vi "HDI Pat Match Full with Move TL.vi"(5 "controller in":refnum<k24>, 11 "error in":errorcluster) -> (4 "In Range?":bool, 8 "x rel move":dbl, 10 "y rel move":dbl, 14 "Vertical vector":dbl[](array[numeric]), 15 "error out":errorcluster)   [LabVIEW 2011]
uses:
  C:/Users/Admin/Desktop/Gantry Code Transfer/source/Code Transfer/Aerotech.A3200.dll
  Aerotech.A3200.dll
  <vilib>/vision/driver/NI_Vision_Acquisition_Software.lvlib
panel:
  out "error out 3":errorcluster
  out "error out 2":errorcluster
  out "Angle Between Lines":dbl
  out "Diagnostic Log":string
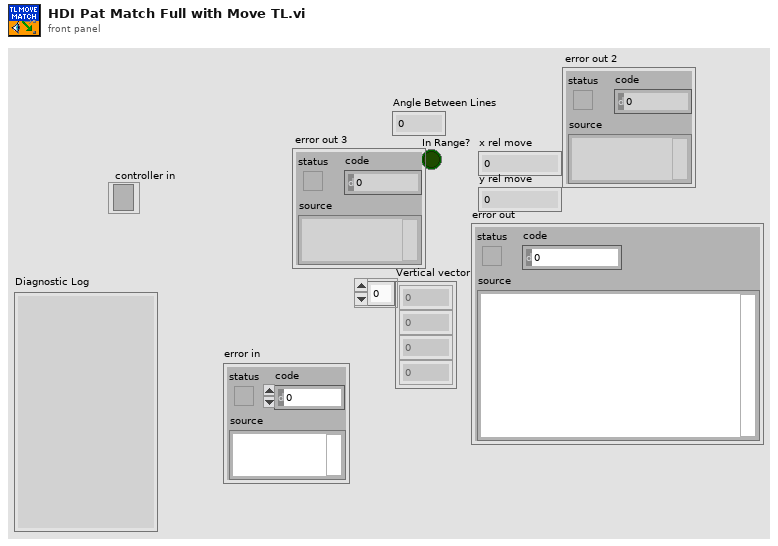
[diagram p1: front panel]
types:
  T1 = typedef "IMAQdx.ctl" = refnum<k21>
  T2 = typedef "IMAQ Image.ctl" = refnum<image>
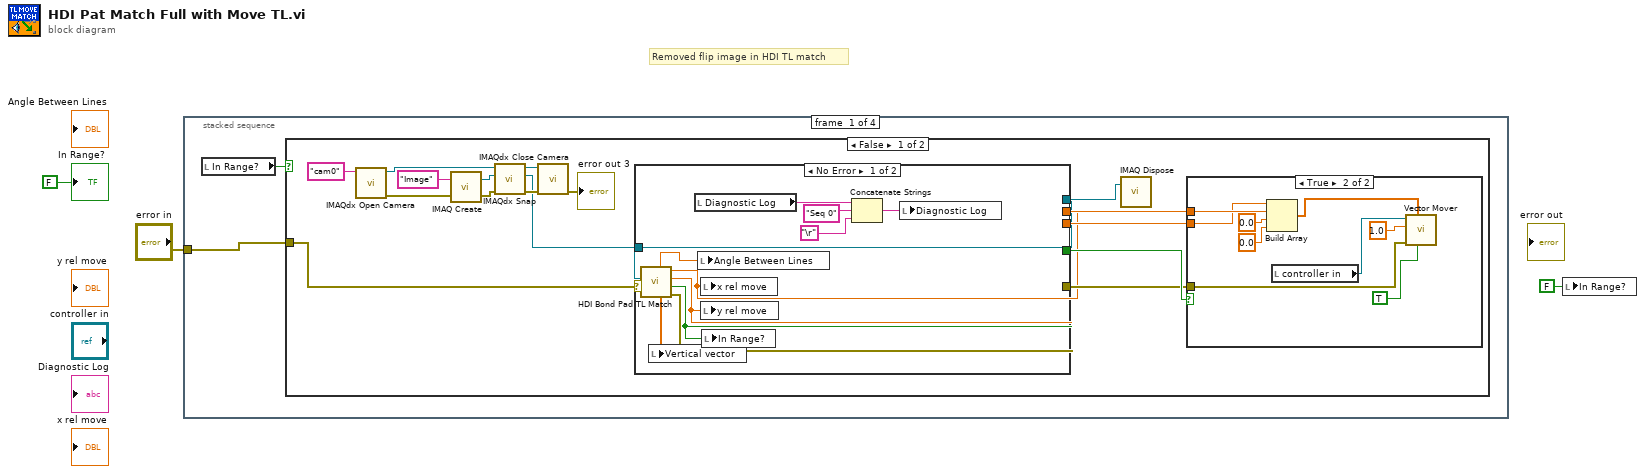
[diagram p0: block diagram]
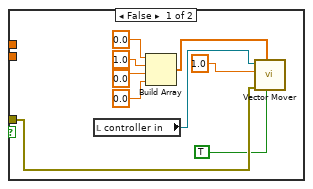
[diagram p2: hidden frame]
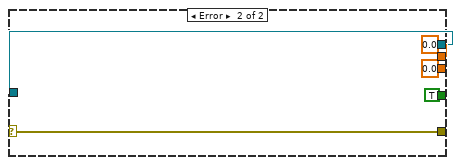
[diagram p3: hidden frame]
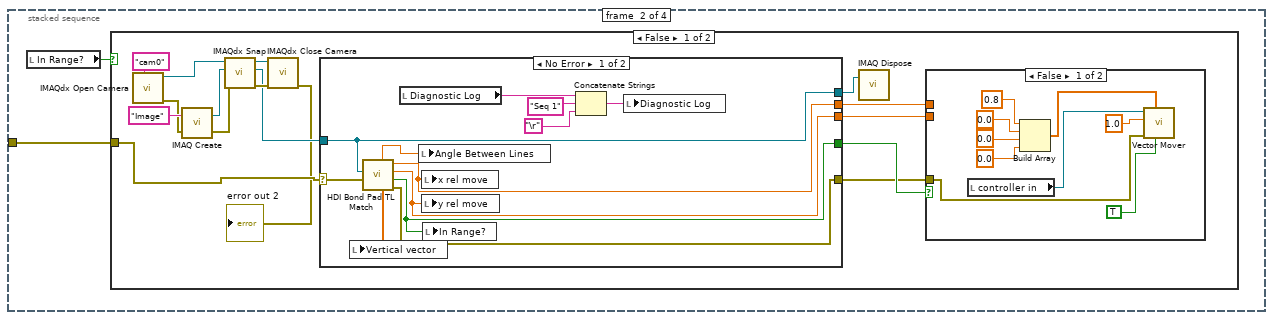
[diagram p5: hidden frame]
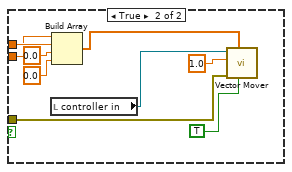
[diagram p6: hidden frame]
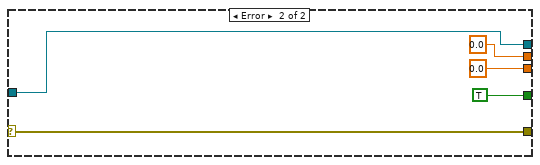
[diagram p7: hidden frame]
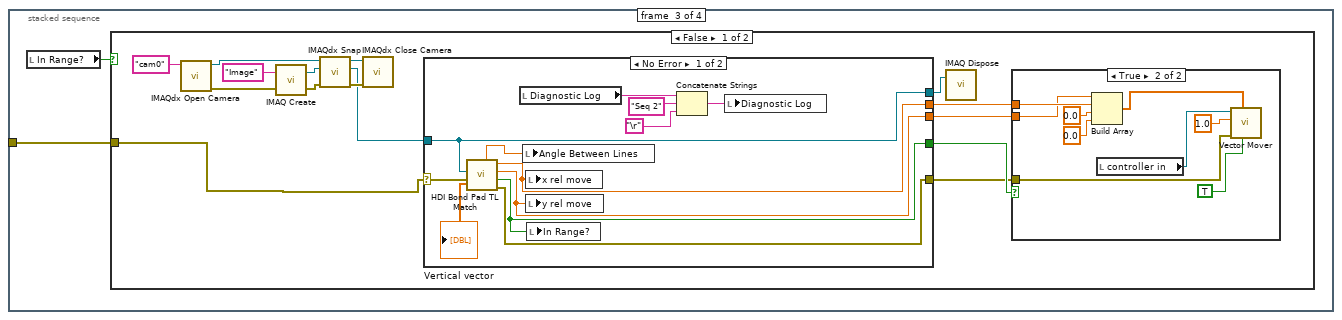
[diagram p9: hidden frame]
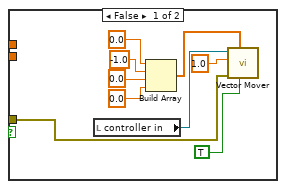
[diagram p10: hidden frame]
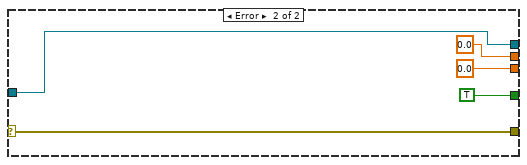
[diagram p11: hidden frame]
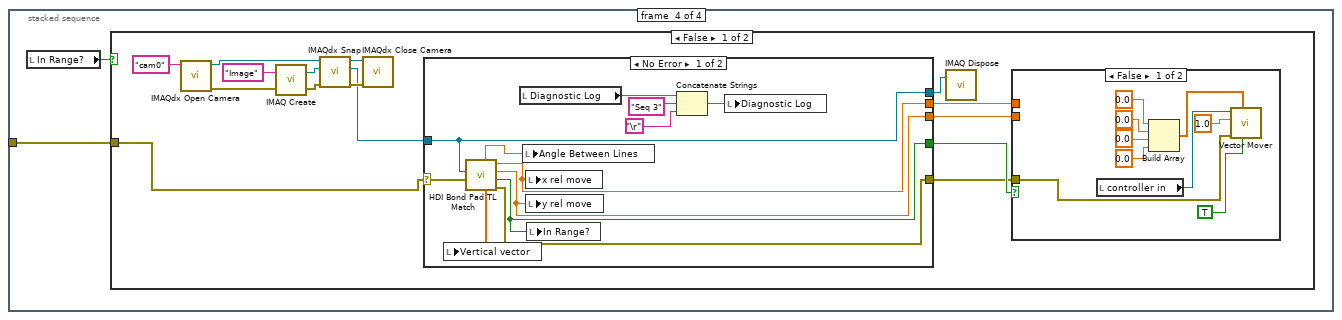
[diagram p13: hidden frame]
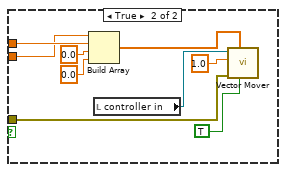
[diagram p14: hidden frame]
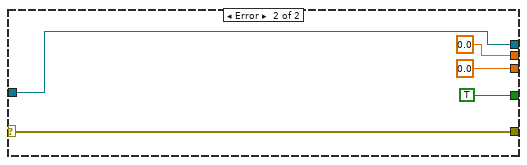
[diagram p15: hidden frame]
diagram:
  # "Removed flip image in HDI TL match"
  n1 = stacked-sequence {
    tunnel: "error in" -> [w4 w57 w110 w162]
    frame #0 {
      n2 = local read "In Range?"() -> (w5:bool)
      n3 = case shown="False" w5 {
        tunnel: w4 -> [w7 _]
        frame False {
          n4 = call <vilib>:"IMAQdx Open Camera.vi"("Session In"="cam0" ("Interface Name")) -> ("error out"=w14:errorcluster, "Session Out"=w9:T1)  [unwired: 9 in]
          n5 = call "IMAQ Create"("Image Name"="Image", "error in (no error)"=w14) -> ("New Image"=w11:T2, "error out"=w10:errorcluster)  [unwired: 3 in]
          n6 = call <vilib>:"IMAQdx Snap.vi"("error in"=w10, "Image In"=w11, "Session In"=w9) -> ("error out"=w12:errorcluster, "Image Out"=w8:T2, "Session Out"=w13:T1)  [unwired: 6 in]
          n7 = call <vilib>:"IMAQdx Close Camera.vi"("error in"=w12, "Session In"=w13) -> ("error out"=→"error out 3":errorcluster)  [unwired: 9 in]
          n8 = case shown="No Error" w7 {
            selector: w7 -> [w50 w56]
            tunnel: [w51 w56] -> w20
            tunnel: [w47 TRUE ("Matched?")] -> w21
            tunnel: [w49 0.0 ("x rel move")] -> w19
            tunnel: [w48 0.0 ("y rel move")] -> w18
            tunnel: w8 -> [w42 w52]
            tunnel: [w42 w52] -> w17
            frame No Error {
              n9 = call "HDI Bond Pad TL Match.vi"("error in (no error)"=w50, "Image Src"=w42) -> ("error out"=w51:errorcluster, "In Range?"=w47:bool, "y rel move"=w48:dbl, "x rel move"=w49:dbl, "Vertical vector"=w40:dbl[], "Angle Between Lines"=w41:dbl)  [unwired: 4 in]
              n10 = local write "Vertical vector"(w40) -> ()
              n11 = local read "Diagnostic Log"() -> (w43:string)
              n12 = local write "Angle Between Lines"(w41) -> ()
              n13 = local write "x rel move"(w49) -> ()
              n14 = local write "y rel move"(w48) -> ()
              n15 = local write "In Range?"(w47) -> ()
              n16 = Concatenate Strings(w43, "Seq 0", "\r") -> (w46:string)
              n17 = local write "Diagnostic Log"(w46) -> ()
            }
            frame Error {
            }
          }
          n18 = call "IMAQ Dispose"("Image"=w17) -> ()  [unwired: 5 in, 1 out]
          n19 = case shown="True" w21 {
            tunnel: w20 -> [w25 w39]
            tunnel: w19 -> [_ w32]
            tunnel: w18 -> [_ w31]
            frame False {
              n20 = local read "controller in"() -> (w24:refnum<k24>)
              n21 = Build Array(0.0 ("element"), 1.0 ("element"), 0.0 ("element"), 0.0 ("element")) -> (w23:dbl[])
              n22 = call "Vector Mover.vi"("Absolute/Relative (F/T)"=TRUE, "Movement Vector"=w23, "error in (no error)"=w25, "Vector Speed"=1.0, "controller in"=w24) -> ()  [unwired: 1 in, 4 out]
            }
            frame True {
              n23 = Build Array(w31, w32, 0.0 ("element"), 0.0 ("element")) -> (w34:dbl[])
              n24 = local read "controller in"() -> (w33:refnum<k24>)
              n25 = call "Vector Mover.vi"("Absolute/Relative (F/T)"=TRUE, "Movement Vector"=w34, "error in (no error)"=w39, "Vector Speed"=1.0, "controller in"=w33) -> ()  [unwired: 1 in, 4 out]
            }
          }
        }
        frame True {
        }
      }
    }
    frame #1 {
      n26 = local read "In Range?"() -> (w58:bool)
      n27 = case shown="False" w58 {
        tunnel: w57 -> [w62 _]
        frame False {
          n28 = call <vilib>:"IMAQdx Open Camera.vi"("Session In"="cam0" ("Interface Name")) -> ("error out"=w60:errorcluster, "Session Out"=w64:T1)  [unwired: 9 in]
          n29 = call "IMAQ Create"("Image Name"="Image", "error in (no error)"=w60) -> ("New Image"=w65:T2, "error out"=w59:errorcluster)  [unwired: 3 in]
          n30 = call <vilib>:"IMAQdx Snap.vi"("error in"=w59, "Image In"=w65, "Session In"=w64) -> ("error out"=w66:errorcluster, "Image Out"=w63:T2, "Session Out"=w67:T1)  [unwired: 6 in]
          n31 = call <vilib>:"IMAQdx Close Camera.vi"("error in"=w66, "Session In"=w67) -> ("error out"=→"error out 2":errorcluster)  [unwired: 9 in]
          n32 = case shown="No Error" w62 {
            selector: w62 -> [w103 w109]
            tunnel: [w104 w109] -> w73
            tunnel: [w100 TRUE ("Matched?")] -> w74
            tunnel: [w102 0.0 ("x rel move")] -> w72
            tunnel: [w101 0.0 ("y rel move")] -> w71
            tunnel: w63 -> [w95 w105]
            tunnel: [w95 w105] -> w70
            frame No Error {
              n33 = call "HDI Bond Pad TL Match.vi"("error in (no error)"=w103, "Image Src"=w95) -> ("error out"=w104:errorcluster, "In Range?"=w100:bool, "y rel move"=w101:dbl, "x rel move"=w102:dbl, "Vertical vector"=w93:dbl[], "Angle Between Lines"=w94:dbl)  [unwired: 4 in]
              n34 = local write "Vertical vector"(w93) -> ()
              n35 = local read "Diagnostic Log"() -> (w96:string)
              n36 = local write "Angle Between Lines"(w94) -> ()
              n37 = local write "x rel move"(w102) -> ()
              n38 = local write "y rel move"(w101) -> ()
              n39 = local write "In Range?"(w100) -> ()
              n40 = Concatenate Strings(w96, "Seq 1", "\r") -> (w99:string)
              n41 = local write "Diagnostic Log"(w99) -> ()
            }
            frame Error {
            }
          }
          n42 = call "IMAQ Dispose"("Image"=w70) -> ()  [unwired: 5 in, 1 out]
          n43 = case shown="False" w74 {
            tunnel: w73 -> [w81 w92]
            tunnel: w72 -> [_ w85]
            tunnel: w71 -> [_ w84]
            frame False {
              n44 = local read "controller in"() -> (w75:refnum<k24>)
              n45 = Build Array(0.8 ("element"), 0.0 ("element"), 0.0 ("element"), 0.0 ("element")) -> (w78:dbl[])
              n46 = call "Vector Mover.vi"("Absolute/Relative (F/T)"=TRUE, "Movement Vector"=w78, "error in (no error)"=w81, "Vector Speed"=1.0, "controller in"=w75) -> ()  [unwired: 1 in, 4 out]
            }
            frame True {
              n47 = local read "controller in"() -> (w87:refnum<k24>)
              n48 = Build Array(w84, w85, 0.0 ("element"), 0.0 ("element")) -> (w86:dbl[])
              n49 = call "Vector Mover.vi"("Absolute/Relative (F/T)"=TRUE, "Movement Vector"=w86, "error in (no error)"=w92, "Vector Speed"=1.0, "controller in"=w87) -> ()  [unwired: 1 in, 4 out]
            }
          }
        }
        frame True {
        }
      }
    }
    frame #2 {
      n50 = local read "In Range?"() -> (w111:bool)
      n51 = case shown="False" w111 {
        tunnel: w110 -> [w112 _]
        frame False {
          n52 = call <vilib>:"IMAQdx Open Camera.vi"("Session In"="cam0" ("Interface Name")) -> ("error out"=w119:errorcluster, "Session Out"=w114:T1)  [unwired: 9 in]
          n53 = call "IMAQ Create"("Image Name"="Image", "error in (no error)"=w119) -> ("New Image"=w116:T2, "error out"=w115:errorcluster)  [unwired: 3 in]
          n54 = call <vilib>:"IMAQdx Snap.vi"("error in"=w115, "Image In"=w116, "Session In"=w114) -> ("error out"=w117:errorcluster, "Image Out"=w113:T2, "Session Out"=w118:T1)  [unwired: 6 in]
          n55 = call <vilib>:"IMAQdx Close Camera.vi"("error in"=w117, "Session In"=w118) -> ()  [unwired: 9 in, 1 out]
          n56 = case shown="No Error" w112 {
            selector: w112 -> [w155 w161]
            tunnel: [w156 w161] -> w125
            tunnel: [w152 TRUE ("Matched?")] -> w126
            tunnel: [w154 0.0 ("x rel move")] -> w124
            tunnel: [w153 0.0 ("y rel move")] -> w123
            tunnel: w113 -> [w147 w157]
            tunnel: [w147 w157] -> w122
            frame No Error {
              n57 = call "HDI Bond Pad TL Match.vi"("error in (no error)"=w155, "Image Src"=w147) -> ("error out"=w156:errorcluster, "In Range?"=w152:bool, "y rel move"=w153:dbl, "x rel move"=w154:dbl, "Vertical vector"=→"Vertical vector":dbl[], "Angle Between Lines"=w146:dbl)  [unwired: 4 in]
              n58 = local read "Diagnostic Log"() -> (w148:string)
              n59 = local write "Angle Between Lines"(w146) -> ()
              n60 = local write "x rel move"(w154) -> ()
              n61 = local write "y rel move"(w153) -> ()
              n62 = local write "In Range?"(w152) -> ()
              n63 = Concatenate Strings(w148, "Seq 2", "\r") -> (w151:string)
              n64 = local write "Diagnostic Log"(w151) -> ()
            }
            frame Error {
            }
          }
          n65 = call "IMAQ Dispose"("Image"=w122) -> ()  [unwired: 5 in, 1 out]
          n66 = case shown="True" w126 {
            tunnel: w125 -> [w133 w144]
            tunnel: w124 -> [_ w137]
            tunnel: w123 -> [_ w136]
            frame False {
              n67 = local read "controller in"() -> (w127:refnum<k24>)
              n68 = Build Array(0.0 ("element"), -1.0 ("element"), 0.0 ("element"), 0.0 ("element")) -> (w130:dbl[])
              n69 = call "Vector Mover.vi"("Absolute/Relative (F/T)"=TRUE, "Movement Vector"=w130, "error in (no error)"=w133, "Vector Speed"=1.0, "controller in"=w127) -> ()  [unwired: 1 in, 4 out]
            }
            frame True {
              n70 = Build Array(w136, w137, 0.0 ("element"), 0.0 ("element")) -> (w139:dbl[])
              n71 = local read "controller in"() -> (w138:refnum<k24>)
              n72 = call "Vector Mover.vi"("Absolute/Relative (F/T)"=TRUE, "Movement Vector"=w139, "error in (no error)"=w144, "Vector Speed"=1.0, "controller in"=w138) -> ()  [unwired: 1 in, 4 out]
            }
          }
        }
        frame True {
        }
      }
    }
    frame #3 {
      n73 = local read "In Range?"() -> (w163:bool)
      n74 = case shown="False" w163 {
        tunnel: w162 -> [w164 _]
        frame False {
          n75 = call <vilib>:"IMAQdx Open Camera.vi"("Session In"="cam0" ("Interface Name")) -> ("error out"=w171:errorcluster, "Session Out"=w166:T1)  [unwired: 9 in]
          n76 = call "IMAQ Create"("Image Name"="Image", "error in (no error)"=w171) -> ("New Image"=w168:T2, "error out"=w167:errorcluster)  [unwired: 3 in]
          n77 = call <vilib>:"IMAQdx Snap.vi"("error in"=w167, "Image In"=w168, "Session In"=w166) -> ("error out"=w169:errorcluster, "Image Out"=w165:T2, "Session Out"=w170:T1)  [unwired: 6 in]
          n78 = call <vilib>:"IMAQdx Close Camera.vi"("error in"=w169, "Session In"=w170) -> ()  [unwired: 9 in, 1 out]
          n79 = case shown="No Error" w164 {
            selector: w164 -> [w207 w213]
            tunnel: [w208 w213] -> w177
            tunnel: [w204 TRUE ("Matched?")] -> w178
            tunnel: [w206 0.0 ("x rel move")] -> w176
            tunnel: [w205 0.0 ("y rel move")] -> w175
            tunnel: w165 -> [w199 w209]
            tunnel: [w199 w209] -> w174
            frame No Error {
              n80 = call "HDI Bond Pad TL Match.vi"("error in (no error)"=w207, "Image Src"=w199) -> ("error out"=w208:errorcluster, "In Range?"=w204:bool, "y rel move"=w205:dbl, "x rel move"=w206:dbl, "Vertical vector"=w197:dbl[], "Angle Between Lines"=w198:dbl)  [unwired: 4 in]
              n81 = local write "Vertical vector"(w197) -> ()
              n82 = local read "Diagnostic Log"() -> (w200:string)
              n83 = local write "Angle Between Lines"(w198) -> ()
              n84 = local write "x rel move"(w206) -> ()
              n85 = local write "y rel move"(w205) -> ()
              n86 = local write "In Range?"(w204) -> ()
              n87 = Concatenate Strings(w200, "Seq 3", "\r") -> (w203:string)
              n88 = local write "Diagnostic Log"(w203) -> ()
            }
            frame Error {
            }
          }
          n89 = call "IMAQ Dispose"("Image"=w174) -> ()  [unwired: 5 in, 1 out]
          n90 = case shown="False" w178 {
            tunnel: w177 -> [w185 w196]
            tunnel: w176 -> [_ w189]
            tunnel: w175 -> [_ w188]
            frame False {
              n91 = local read "controller in"() -> (w179:refnum<k24>)
              n92 = Build Array(0.0 ("element"), 0.0 ("element"), 0.0 ("element"), 0.0 ("element")) -> (w182:dbl[])
              n93 = call "Vector Mover.vi"("Absolute/Relative (F/T)"=TRUE, "Movement Vector"=w182, "error in (no error)"=w185, "Vector Speed"=1.0, "controller in"=w179) -> ()  [unwired: 1 in, 4 out]
            }
            frame True {
              n94 = Build Array(w188, w189, 0.0 ("element"), 0.0 ("element")) -> (w191:dbl[])
              n95 = local read "controller in"() -> (w190:refnum<k24>)
              n96 = call "Vector Mover.vi"("Absolute/Relative (F/T)"=TRUE, "Movement Vector"=w191, "error in (no error)"=w196, "Vector Speed"=1.0, "controller in"=w190) -> ()  [unwired: 1 in, 4 out]
            }
          }
        }
        frame True {
        }
      }
    }
  }
  n97 = local write "In Range?"(FALSE ("In Range?")) -> ()
  "In Range?" <- FALSE ("In Range?")
